vi "InvokePPP.vi"(8 "error in (no error)":errorcluster, 10 "PPP_parameters":T1={"product"="C30L", "printer"="DL_1", "printhead"=enum."1", "material"="C30L", "weight"=0.0898, "density"=1.0, "overprint"=1.15, "print_wt_multiplier"=5.0, "num_of_drops"=735957, "gs_source"="DB", "gs_val_file"=path "None", "zone_compensation"=TRUE, "zone_comp_file"=path "compensation_zone_list2.csv", "bitmap"=path "WBG_images/DL_1_C30L.bmp", "save_gs_img"=TRUE, "dithered_save_path"=path "cwd/Dithered_images", "gs_save_path"=path "cwd/Saved_GS_images", "rotation"=TRUE, "driver"="SQL Server", "server"="tt-local.digilens.com", "database"="ToolTrack", "user"="tooltrack-user", "password"="DigiLens_rEAd_passwrd"}, 11 "Py Session":refnum<k35>) -> (0 "error out":errorcluster, 2 "Cluster":cluster{"Success":bool, "Status":string}, 3 "Py Session out":refnum<k35>)   [LabVIEW 2022 SP3, in "DLP2.lvclass"]
uses:
  DLP2.lvclass
  DataTypes/PPP_Python--cluster.ctl
  TopLevel/Typedefs/PrinterHeads--Enum.ctl
panel:
  out "return code":i32
  out "Sys Exec Command":string
  # "python PPP_app_CLI.py -t C30L -p DL_1 -ph 1 -m C30L -w 0.0898 -d 1.00 -o 1.15 -x 5 -n 735957 -f DB -l None -z True -c compensation_zone_list2.csv -b WBG_images\\DL_1_C30L.bmp -r True -s cwd\\Dithered_images -g cwd\\Saved_GS_images -ro True -dr \"SQL Server\" -se tt-local.digilens.com -db ToolTrack -u tooltrack-user -pa DigiLens_rEAd_passwrd"
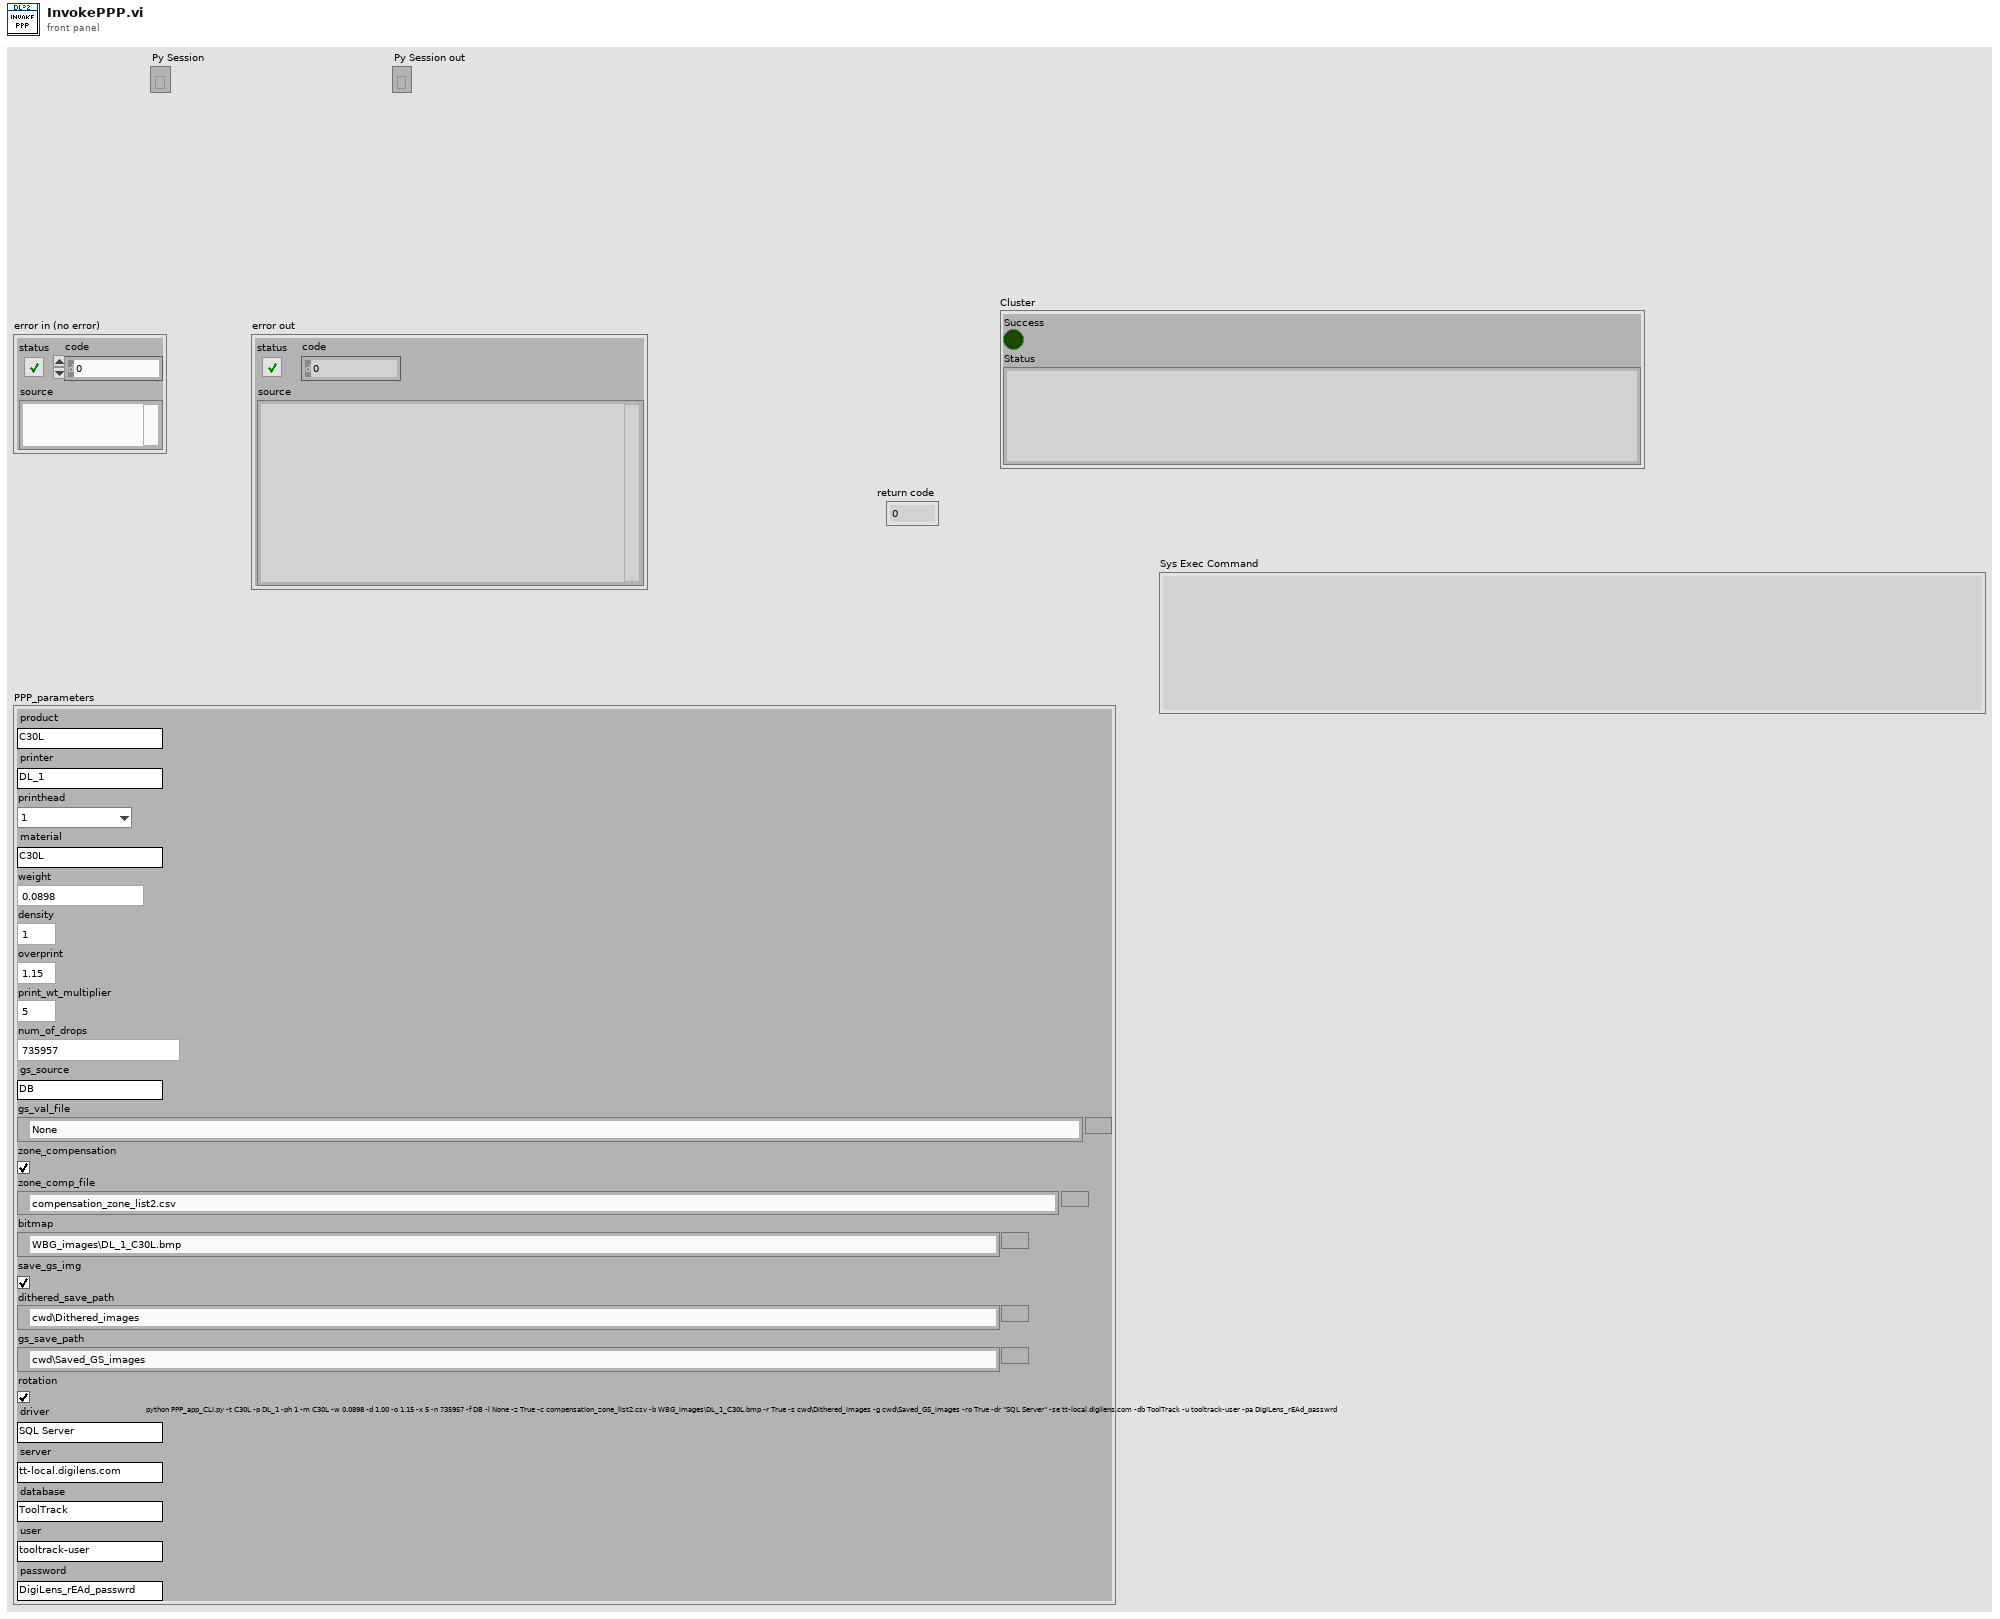
[diagram p1: front panel]
types:
  T1 = typedef "PPP_Python--cluster.ctl" = cluster{"product":string, "printer":string, "printhead":T2, "material":string, "weight":dbl, "density":dbl, "overprint":dbl, "print_wt_multiplier":dbl, "num_of_drops":i32, "gs_source":string, "gs_val_file":path, "zone_compensation":bool, "zone_comp_file":path, "bitmap":path, "save_gs_img":bool, "dithered_save_path":path, "gs_save_path":path, "rotation":bool, "driver":string, "server":string, "database":string, "user":string, "password":string}
  T2 = typedef "PrinterHeads--Enum.ctl" = enum16{"-1", "1", "2", "3", "4", "5", "6"}
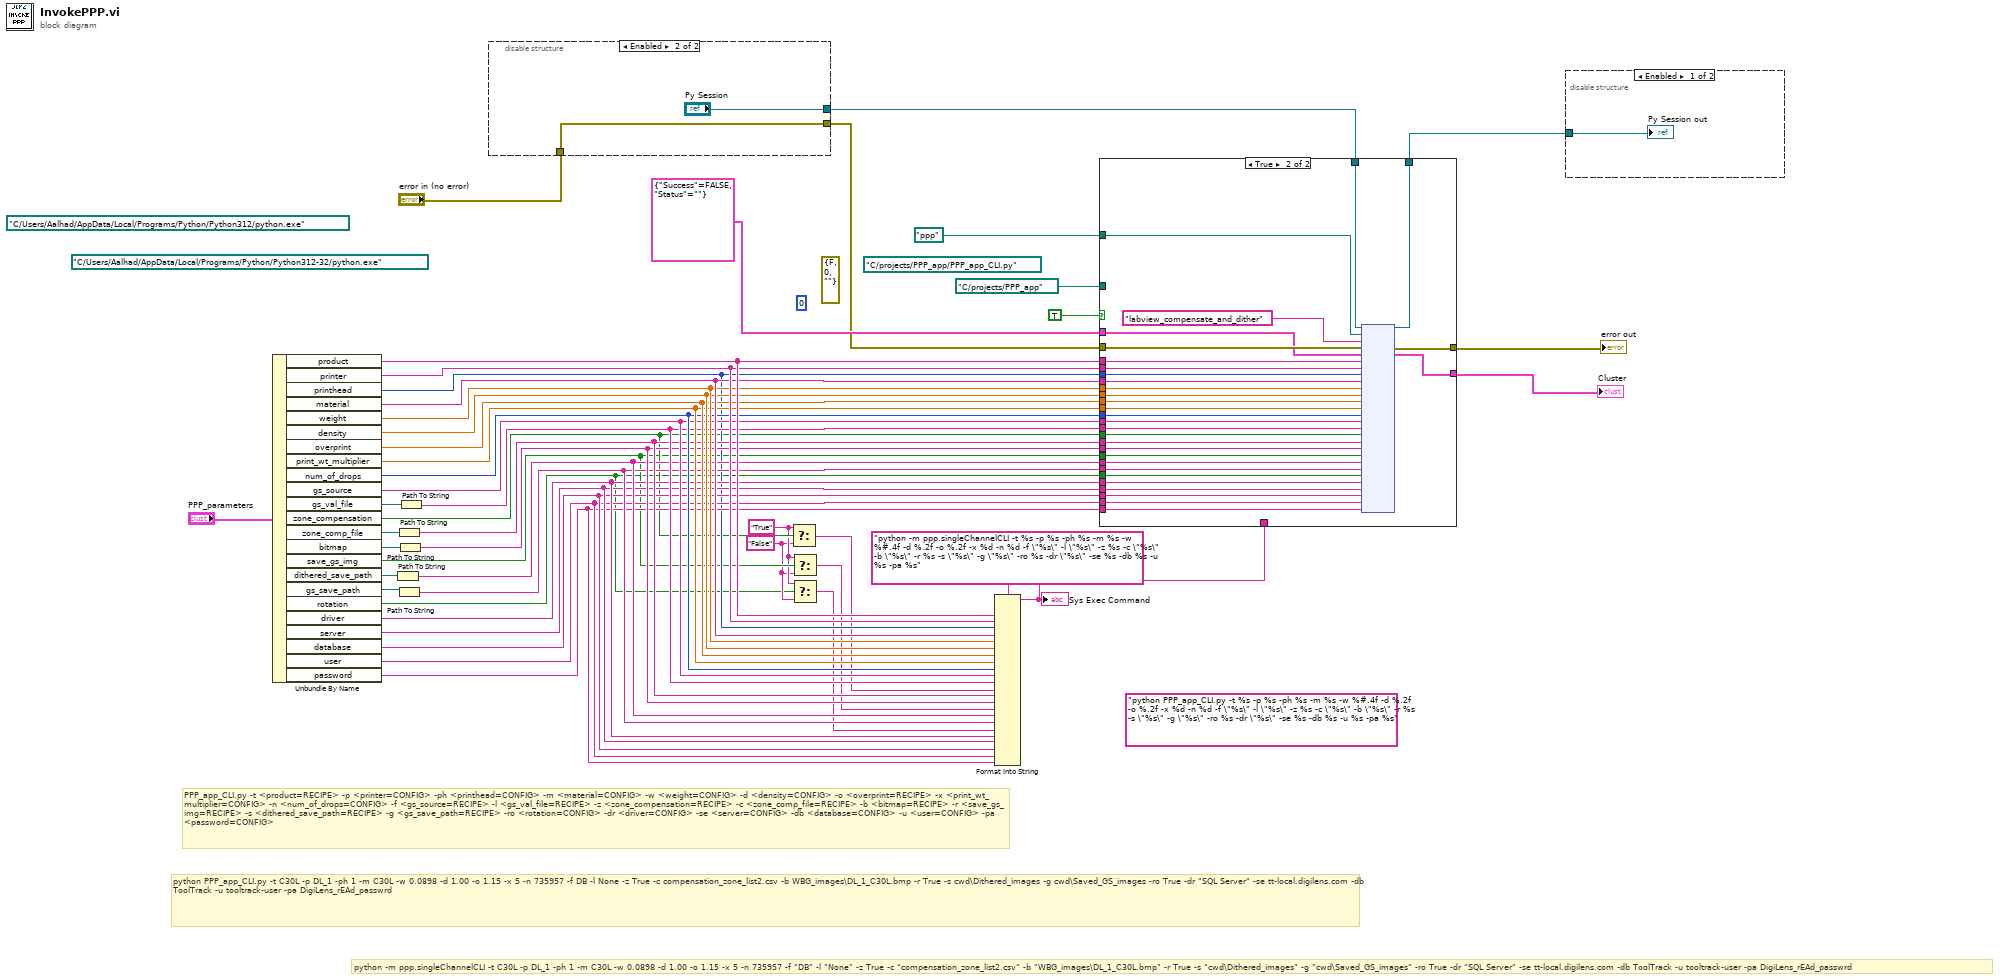
[diagram p0: block diagram]
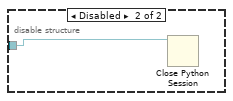
[diagram p2: hidden frame]
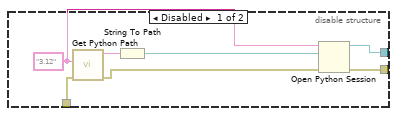
[diagram p3: hidden frame]
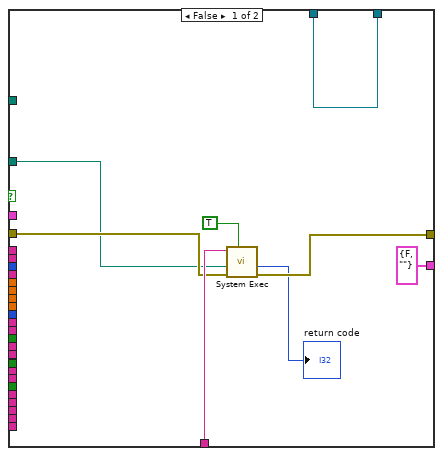
[diagram p4: hidden frame]
diagram:
  (unwired) errorcluster {"status"=FALSE, "code"=0, "source"=""} ("error out")
  (unwired) 0
  (unwired) "python PPP_app_CLI.py -t %s -p %s -ph %s -m %s -w %#.4f -d %.2f -o %.2f -x %d -n %d -f \"%s\" -l \"%s\" -z %s -c \"%s\" -b \"%s\" -r %s -s \"%s\" -g \"%s\" -ro %s -dr \"%s\" -se %s -db %s -u %s -pa %s" ("format string")
  (unwired) path "C:/projects/PPP_app/PPP_app_CLI.py"
  w12 = "False" ("f")
  w13 = "True"
  (unwired) path "C:/Users/Aalhad/AppData/Local/Programs/Python/Python312-32/python.exe" ("Python path")
  (unwired) path "C:/Users/Aalhad/AppData/Local/Programs/Python/Python312/python.exe" ("Python path")
  # "python -m ppp.singleChannelCLI -t C30L -p DL_1 -ph 1 -m C30L -w 0.0898 -d 1.00 -o 1.15 -x 5 -n 735957 -f \"DB\" -l \"None\" -z True -c \"compensation_zone_list2.csv\" -b \"WBG_images\\DL_1_C30L.bmp\" -r True -s \"cwd\\Dithered_images\" -g \"cwd\\Saved_GS_images\" -ro True -dr \"SQL Server\" -se tt-local.digilens.com -db ToolTrack -u tooltrack-user -pa DigiLens_rEAd_passwrd"
  # "python PPP_app_CLI.py -t C30L -p DL_1 -ph 1 -m C30L -w 0.0898 -d 1.00 -o 1.15 -x 5 -n 735957 -f DB -l None -z True -c compensation_zone_list2.csv -b WBG_images\\DL_1_C30L.bmp -r True -s cwd\\Dithered_images -g cwd\\Saved_GS_images -ro True -dr \"SQL Server\" -se tt-local.digilens.com -db ToolTrack -u tooltrack-user -pa DigiLens_rEAd_passwrd"
  # "PPP_app_CLI.py -t <product=RECIPE> -p <printer=CONFIG> -ph <printhead=CONFIG> -m <material=CONFIG> -w <weight=CONFIG> -d <density=CONFIG> -o <overprint=RECIPE> -x <print_wt_multiplier=CONFIG> -n <num_of_drops=CONFIG> -f <gs_source=RECIPE> -l <gs_val_file=RECIPE> -z <zone_compensation=RECIPE> -c <zone_comp_file=RECIPE> -b <bitmap=RECIPE> -r <save_gs_img=RECIPE> -s <dithered_save_path=RECIPE> -g <gs_save_path=RECIPE> -ro <rotation=CONFIG> -dr <driver=CONFIG> -se <server=CONFIG> -db <database=CONFIG> -u <user=CONFIG> -pa <password=CONFIG>"
  n1 = Unbundle By Name("PPP_parameters") -> ("product"=w37:string, "printer"=w36:string, "printhead"=w18:T2, "material"=w35:string, "weight"=w34:dbl, "density"=w33:dbl, "overprint"=w32:dbl, "print_wt_multiplier"=w31:dbl, "num_of_drops"=w30:i32, "gs_source"=w29:string, "gs_val_file"=w43:path, "zone_compensation"=w17:bool, "zone_comp_file"=w42:path, "bitmap"=w41:path, "save_gs_img"=w15:bool, "dithered_save_path"=w40:path, "gs_save_path"=w39:path, "rotation"=w11:bool, "driver"=w23:string, "server"=w22:string, "database"=w21:string, "user"=w20:string, "password"=w19:string)
  n2 = Path To String(path=w40) -> (string=w25:string)
  n3 = Path To String(path=w42) -> (string=w27:string)
  n4 = Path To String(path=w39) -> (string=w24:string)
  n5 = Path To String(path=w41) -> (string=w26:string)
  n6 = Path To String(path=w43) -> (string=w28:string)
  n7 = disable-structure shown="Enabled" {
    disable-tunnel: [w50 "Py Session"] -> w5
    disable-tunnel: [w49 w54] -> w2
    disable-tunnel: "error in (no error)" -> [w47 w54]
    frame Disabled {
      w51 = "3.12" ("Python Rev Key")
      n8 = call "Get Python Path.vi"("error in (no error)"=w47, "Python Rev Key"=w51) -> ("error out"=w48:errorcluster, "Python.exe path"=w53:string)  [unwired: 8 in]
      n9 = String To Path(string=w53) -> (path=w52:path)
      n10 = Open Python Session(python version=w51, python path=w52, 3:w48) -> (session out=w50:refnum<k35>, error out=w49:errorcluster)
    }
    frame Enabled {
    }
  }
  n11 = Select(t=w13, s=w17, f=w12) -> (s? t:f=w16:string)
  n12 = Select(t=w13, s=w15, f=w12) -> (s? t:f=w14:string)
  n13 = Select(t=w13, s=w11, f=w12) -> (s? t:f=w10:string)
  n14 = Format Into String(format string="python -m ppp.singleChannelCLI -t %s -p %s -ph %s -m %s -w %#.4f -d %.2f -o %.2f -x %d -n %d -f \"%s\" -l \"%s\" -z %s -c \"%s\" -b \"%s\" -r %s -s \"%s\" -g \"%s\" -ro %s -dr \"%s\" -se %s -db %s -u %s -pa %s", w37, w36, w18, w35, w34, w33, w32, w31, w30, w29, w28, w16, w27, w26, w14, w25, w24, w10, w23, w22, w21, w20, w19) -> (resulting string=w9:string)  [unwired: 2 in, 1 out]
  "Sys Exec Command" <- w9
  n15 = case shown="True" TRUE {
    tunnel: [w63 w94] -> w46
    tunnel: w5 -> [w63 w93]
    tunnel: w2 -> [w61 w92]
    tunnel: [w60 w91] -> w45
    tunnel: w37 -> [_ w90]
    tunnel: w36 -> [_ w89]
    tunnel: w35 -> [_ w88]
    tunnel: w34 -> [_ w87]
    tunnel: w33 -> [_ w86]
    tunnel: w32 -> [_ w85]
    tunnel: w31 -> [_ w84]
    tunnel: w30 -> [_ w83]
    tunnel: w29 -> [_ w82]
    tunnel: w28 -> [_ w81]
    tunnel: w27 -> [_ w80]
    tunnel: w26 -> [_ w79]
    tunnel: w25 -> [_ w78]
    tunnel: w24 -> [_ w77]
    tunnel: w23 -> [_ w76]
    tunnel: w22 -> [_ w75]
    tunnel: w21 -> [_ w74]
    tunnel: w20 -> [_ w73]
    tunnel: w19 -> [_ w72]
    tunnel: w18 -> [_ w71]
    tunnel: w17 -> [_ w70]
    tunnel: w15 -> [_ w69]
    tunnel: w11 -> [_ w68]
    tunnel: w9 -> [w62 _]
    tunnel: path "ppp" -> [_ w67]
    tunnel: path "C:/projects/PPP_app" ("working directory") -> [w58 _]
    tunnel: [cluster{"Error":bool, "Status":string} {"Error"=FALSE, "Status"=""} w66] -> w3
    tunnel: cluster{"Success":bool, "Status":string} {"Success"=FALSE, "Status"=""} -> [_ w65]
    frame False {
      n16 = call <vilib>:"System Exec.vi"("wait until completion? (T)"=TRUE, "error in (no error)"=w61, "working directory"=w58, "command line"=w62) -> ("error out"=w60:errorcluster, "return code"=→"return code":i32)  [unwired: 4 in, 2 out]
    }
    frame True {
      n17 = node(w93, w67, "labview_compensate_and_dither" ("function name"), w92, w65, w90, w89, w71, w88, w87, w86, w85, w84, w83, w82, w81, w70, w80, w79, w69, w78, w77, w68, w76, w75, w74, w73, w72) -> (w94:refnum<k35>, w91:errorcluster, w66:cluster{"Success":bool, "Status":string})  [unwired: 23 in, 2 out]
    }
  }
  "error out" <- w45
  "Cluster" <- w3
  n18 = disable-structure shown="Enabled" {
    disable-tunnel: w46 -> [w95 w96]
    frame Enabled {
      "Py Session out" <- w95
    }
    frame Disabled {
      n19 = Close Python Session(session in=w96) -> ()  [unwired: 1 in, 1 out]
    }
  }
